vi "setShutdownEvent.vi"(10 "ShutdownEvent":refnum<user-event>, 11 "UserEvents in":refnum<class "UserEvents.lvclass">) -> (3 "UserEvents out":refnum<class "UserEvents.lvclass">)   [LabVIEW 2016, in "UserEvents.lvclass"]
uses:
  UserEvents.lvclass
  Types/ShutdownEvent.ctl
  UserEvents.lvclass/UserEvents.ctl
  Types/M1M3SupportTypes.lvlib
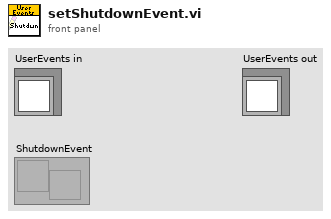
[diagram p1: front panel]
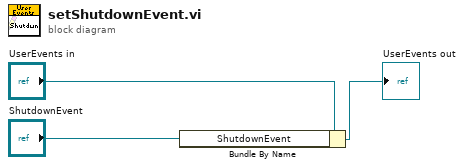
[diagram p0: block diagram]
diagram:
  n1 = Bundle By Name(cluster="UserEvents in", "ShutdownEvent"="ShutdownEvent") -> (→"UserEvents out":refnum<class "UserEvents.lvclass">)
